vi "Run.vi"(8 "error in (no error)":errorcluster, 9 "Time Ratio used":dbl, 10 "Maze (0: Empty, -1: Enemy. >0: Teammate":i32[][](array[numeric]), 11 "TeamEffort in":refnum<class "TeamEffort.lvclass">) -> (0 "error out":errorcluster, 1 "Direction":T1, 2 "Action":T2, 3 "TeamEffort out":refnum<class "TeamEffort.lvclass">, 4 "Replicated":refnum<class "Square.lvclass">)   [LabVIEW 2014, in "TeamEffort.lvclass"]
uses:
  Square/Shawn/TeamEffort/TeamEffort.lvclass
  private/Player Cluster.ctl
  private/Grid Cluster.ctl
  SquareBattle Arena/Action Enum.ctl
  SquareBattle Arena/SquareBattle Arena.lvclass
  SquareBattle Arena/Direction Enum.ctl
  Square/Square.lvclass
panel:
  # "NOTICE - YOU MUST NOT REMOVE THIS NOTICE. PER THE FOLLOWING LICENSE, YOU MAY REPRODUCE THIS SOFTWARE PROVIDED YOU FOLLOW THE TERMS\nOF THE LICENSE.\n\n---BEGIN BSD LICENSE (http://opensource.org/licenses/BSD-2-Clause)---\nCopyright (c) 2015, Endigit, Inc. <robert@endigit.com>\nAll rights reserved.\n\nRedistribution and use in source and binary forms, with or without modification, are permitted provided that the following conditions are met:\n\n1. Redistributions of source code must retain the above copyright notice, this list of conditions and the following disclaimer.\n\n2. Redistributions in binary form must reproduce the above copyright notice, this list of conditions and the following disclaimer in the documentation and/or other \nmaterials provided with the distribution.\n\nTHIS SOFTWARE IS PROVIDED BY THE COPYRIGHT HOLDERS AND CONTRIBUTORS \"AS IS\" AND ANY EXPRESS OR IMPLIED WARRANTIES, INCLUDING, BUT NOT \nLIMITED TO, THE IMPLIED WARRANTIES OF MERCHANTABILITY AND FITNESS FOR A PARTICULAR PURPOSE ARE DISCLAIMED. IN NO EVENT SHALL THE COPYRIGHT \nHOLDER OR CONTRIBUTORS BE LIABLE FOR ANY DIRECT, INDIRECT, INCIDENTAL, SPECIAL, EXEMPLARY, OR CONSEQUENTIAL DAMAGES (INCLUDING, BUT NOT \nLIMITED TO, PROCUREMENT OF SUBSTITUTE GOODS OR SERVICES; LOSS OF USE, DATA, OR PROFITS; OR BUSINESS INTERRUPTION) HOWEVER CAUSED AND ON \nANY THEORY OF LIABILITY, WHETHER IN CONTRACT, STRICT LIABILITY, OR TORT (INCLUDING NEGLIGENCE OR OTHERWISE) ARISING IN ANY WAY OUT OF THE USE \nOF THIS SOFTWARE, EVEN IF ADVISED OF THE POSSIBILITY OF SUCH DAMAGE.\n---END BSD LICENSE---"
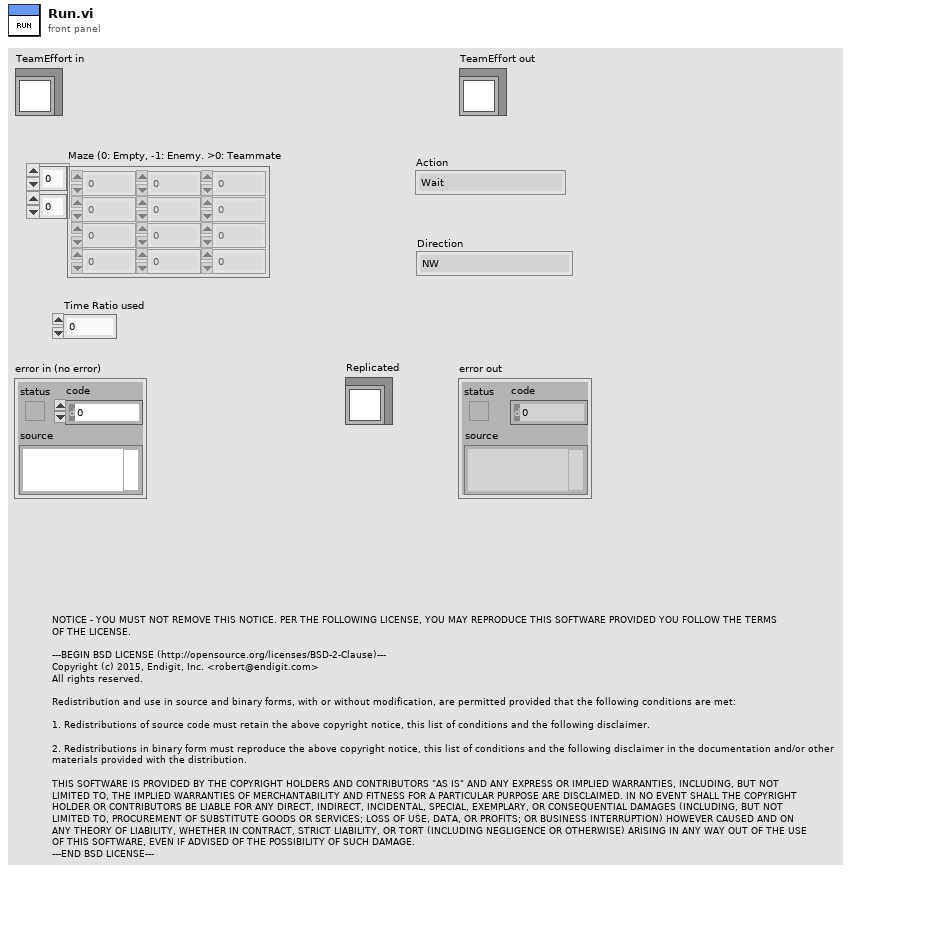
[diagram p1: front panel]
types:
  T1 = typedef "SquareBattle Arena.lvlib/SquareBattle Arena.lvclass/Direction Enum.ctl" = enum16{"NW", "N", "NE", "E", "SE", "S", "SW", "W"}
  T2 = typedef "SquareBattle Arena.lvlib/SquareBattle Arena.lvclass/Action Enum.ctl" = enum16{"Wait", "Move", "Attack", "Replicate"}
  T3 = typedef "TeamEffort.lvclass/Grid Cluster.ctl" = cluster{"p[x][y]":i32[][], "Move Count":i32, "Info[p]":T4[]}
  T4 = typedef "TeamEffort.lvclass/Player Cluster.ctl" = cluster{"Player #":i32, "Exp. Move":i32, "X":i16, "Y":i16, "Action":T2, "Direction":T1, "Moved?":bool}
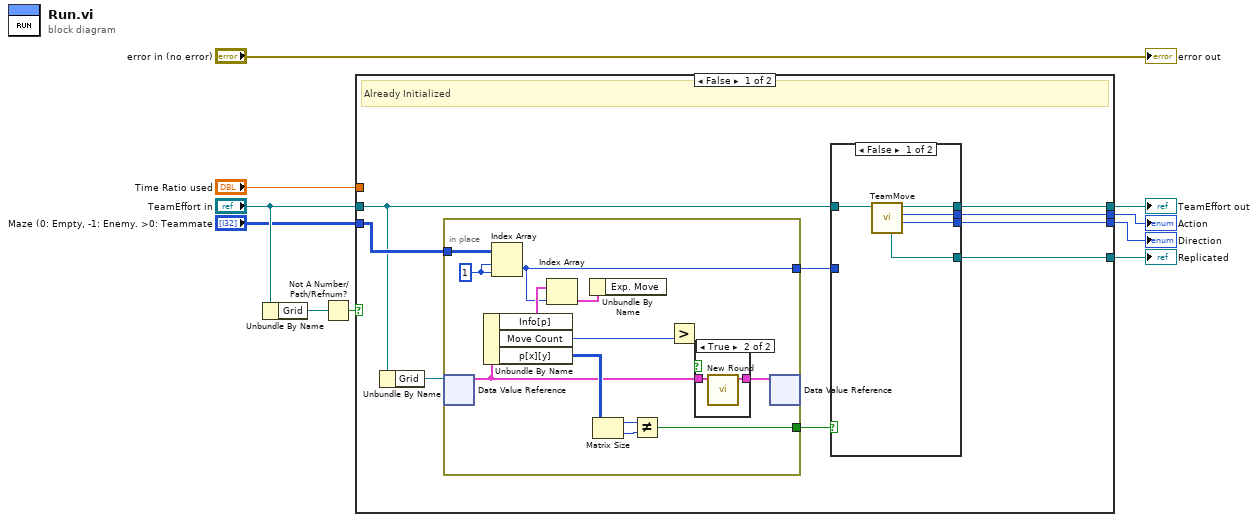
[diagram p0: block diagram]
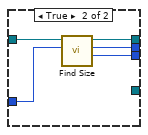
[diagram p3: hidden frame]
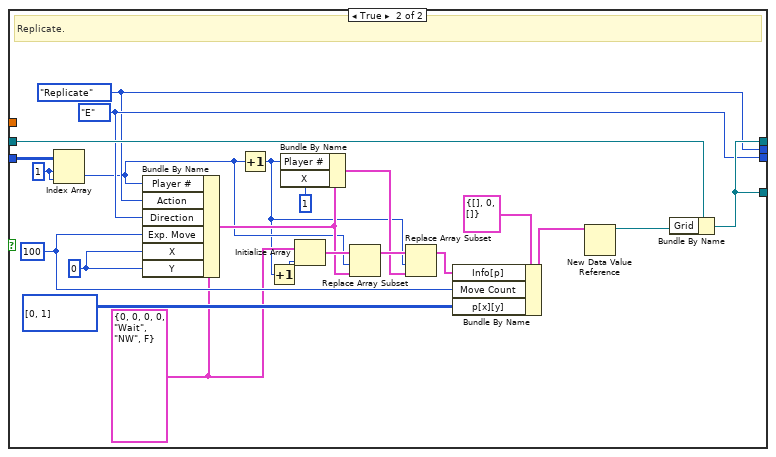
[diagram p4: hidden frame]
diagram:
  n1 = Unbundle By Name("TeamEffort in") -> ("Grid"=w10:refnum<data-value>)
  n2 = Not A Number/Path/Refnum?(number/path/refnum=w10) -> (NaN/Path/Refnum?=w9:bool)
  n3 = case shown="False" w9 {
    tunnel: "TeamEffort in" -> [w16 w67]
    tunnel: [w11 w62] -> w7
    tunnel: [w14 w58] -> w6
    tunnel: [w13 w59] -> w5
    tunnel: "Maze (0: Empty, -1: Enemy. >0: Teammate" -> [w19 w65]
    tunnel: [w12 w62] -> w2
    tunnel: "Time Ratio used" -> [_ _]
    frame False {
      # "Already Initialized"
      n4 = Unbundle By Name(w16) -> ("Grid"=w17:refnum<data-value>)
      n5 = in-place {
        in-place-border: w19 -> [w29]
        in-place-border: [w25] -> w18
        in-place-border: [w20] -> w15
        w28 = 1
        n6 = in-place-dvr #1(w17) -> (w24:T3)  [unwired: 1 out]
        n7 = Unbundle By Name(w24) -> ("Info[p]"=w22:T4[], "Move Count"=w26:i32, "p[x][y]"=w30:i32[][])
        n8 = Index Array(array=w29, index (row)=w28, index (col)=w28) -> (element=w20:i32)
        n9 = Index Array(array=w22, index=w20) -> (element=w21:T4)
        n10 = Unbundle By Name(w21) -> ("Exp. Move"=w27:i32)
        n11 = Matrix Size(0:w30) -> (1:w31:i32, 2:w32:i32)
        n12 = Not Equal?(x=w31, y=w32) -> (x != y?=w25:bool)
        n13 = Greater?(y=w26) -> ()  [unwired: 1 in, 1 out]
        n14 = case shown="True" {
          selector: _ -> [_ _]
          tunnel: w24 -> [w33 w35]
          tunnel: [w33 w34] -> w23
          frame False {
          }
          frame True {
            n15 = call "New Round.vi"("Grid"=w35) -> ("Grid out"=w34:T3)  [unwired: 9 in, 1 out]
          }
        }
        n16 = in-place-dvr #1(w23) -> ()  [unwired: 2 out]
      }
      n17 = case shown="False" w18 {
        tunnel: w16 -> [w40 w45]
        tunnel: w15 -> [_ w44]
        tunnel: [w39 w43] -> w12
        tunnel: [w38 w42] -> w14
        tunnel: [w37 w41] -> w13
        tunnel: [w36 _] -> w11
        frame False {
          n18 = call-dynamic "TeamMove.vi"("TeamEffort in"=w40) -> ("Direction"=w37:T1, "Action"=w38:T2, "TeamEffort out"=w39:refnum<class "TeamEffort.lvclass">, "Replicated"=w36:refnum<class "Square.lvclass">)  [unwired: 6 in, 1 out]
        }
        frame True {
          n19 = call "Find Size.vi"("p"=w44, "TeamEffort in"=w45) -> ("Direction"=w41:T1, "Action"=w42:T2, "TeamEffort out"=w43:refnum<class "TeamEffort.lvclass">)  [unwired: 6 in, 1 out]
        }
      }
    }
    frame True {
      w60 = i16 0 ("index (row)")
      w64 = 1 ("index (row)")
      w56 = T4 {"Player #"=0, "Exp. Move"=0, "X"=0, "Y"=0, "Action"=enum."Wait", "Direction"=enum."NW", "Moved?"=FALSE} ("Player Info")
      w59 = Direction_Enum."E" ("Direction")
      w58 = Action_Enum."Replicate" ("Action")
      w61 = 100 ("Move Count")
      # "Replicate."
      n20 = Index Array(array=w65, index (row)=w64, index (col)=w64) -> (element=w49:i32)
      n21 = Bundle By Name(cluster=w56, "Player #"=w49, "Action"=w58, "Direction"=w59, "Exp. Move"=w61, "X"=w60, "Y"=w60) -> (w51:T4)
      n22 = Increment(x=w49) -> (x+1=w48:i32)
      n23 = Increment(x=w48) -> (x+1=w50:i32)
      n24 = Bundle By Name(cluster=w51, "Player #"=w48, "X"=i16 1 ("index (row)")) -> (w52:T4)
      n25 = Initialize Array(w56, w50) -> (w55:T4[])
      n26 = Replace Array Subset(array=w55, new element=w51, index=w49) -> (w54:T4[])
      n27 = Replace Array Subset(array=w54, new element=w52, index=w48) -> (w53:T4[])
      n28 = Bundle By Name(cluster=T3 {"p[x][y]"=[], "Move Count"=0, "Info[p]"=[]} ("Grid"), "Info[p]"=w53, "Move Count"=w61, "p[x][y]"=i32[][] [[0, 1]]) -> (w47:T3)
      n29 = New Data Value Reference(data value=w47) -> (data value reference=w46:refnum<data-value>)  [unwired: 1 in, 1 out]
      n30 = Bundle By Name(cluster=w67, "Grid"=w46) -> (w62:refnum<class "TeamEffort.lvclass">)
    }
  }
  "TeamEffort out" <- w2
  "Action" <- w6
  "Direction" <- w5
  "Replicated" <- w7
  "error out" <- "error in (no error)"
